vi "mean_squared_error.vi"(1 "Array":dbl[](array[numeric])) -> (0 "Mean Squared Error":dbl)   [LabVIEW 2017]
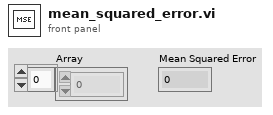
[diagram p1: front panel]
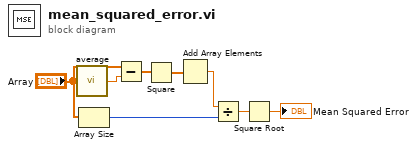
[diagram p0: block diagram]
diagram:
  n1 = call "average.vi"("Array"="Array") -> ("Average"=w1:dbl)
  n2 = Array Size(array="Array") -> (size(s)=w6:i32)
  n3 = Subtract(x="Array", y=w1) -> (x-y=w2:dbl[])
  n4 = Square(x=w2) -> (x^2=w3:dbl[])
  n5 = Add Array Elements(numeric array=w3) -> (sum=w4:dbl)
  n6 = Divide(x=w4, y=w6) -> (x/y=w7:dbl)
  n7 = Square Root(x=w7) -> (sqrt(x)=→"Mean Squared Error":dbl)
